vi "List Permanent Variables.vi"(8 "error in (no error)":errorcluster, 11 "CSM-Static-Variable-Manager in":refnum<class "CSM-Static-Variable-Manager.lvclass">) -> (0 "error out":errorcluster, 1 "Permanent Variables":string[](array[string]), 3 "CSM-Static-Variable-Manager out":refnum<class "CSM-Static-Variable-Manager.lvclass">)   [LabVIEW 2017, in "INI-Static-Variable-Support.lvlib" / "CSM-Static-Variable-Manager.lvclass"]
uses:
  CSM-Static-Variable-Manager.lvclass
  CSM-Static-Variable-Manager.lvclass/CSM-Static-Variable-Manager.ctl
  LabVIEW-Config/LabVIEW-Config.lvclass
  <userlib>/_NEVSTOP/Communicable State Machine(CSM)/addons/API-String-Arugments-Support/API String Arguments Support.lvlib
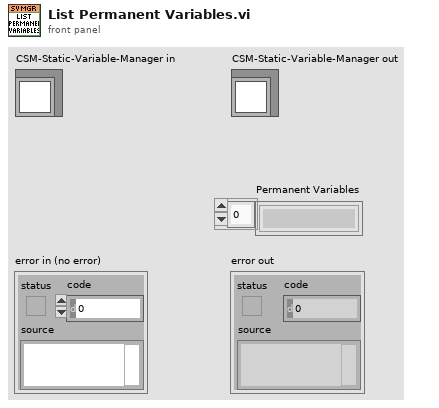
[diagram p1: front panel]
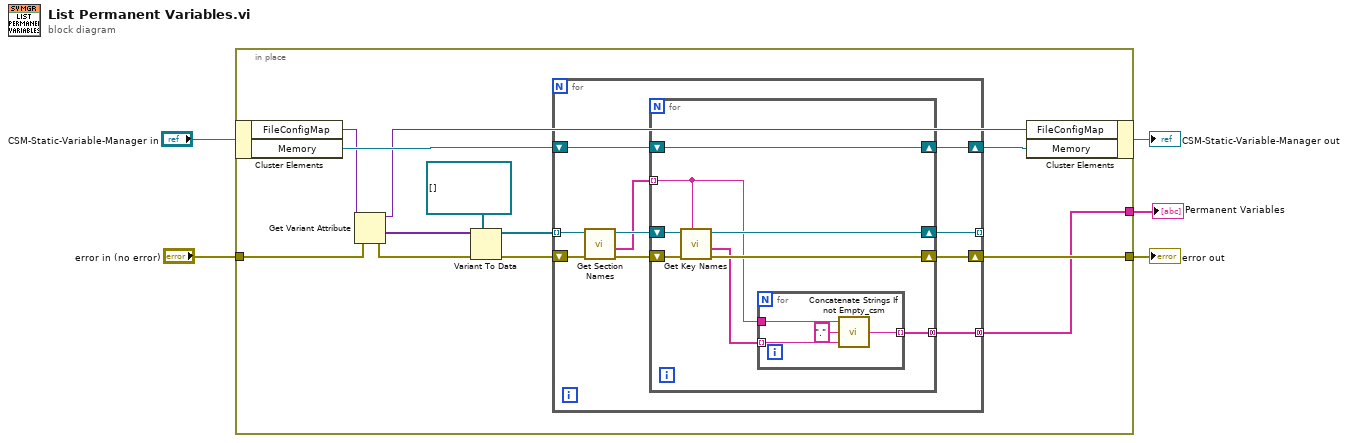
[diagram p0: block diagram]
diagram:
  n1 = in-place {
    in-place-border: "error in (no error)" -> [w12]
    in-place-border: [w8] -> w2
    in-place-border: [w6] -> w1
    n2 = in-place-cluster #1("CSM-Static-Variable-Manager in") -> ("FileConfigMap"=w15:variant, "Memory"=w17:refnum<class "LabVIEW-Config.lvclass">)
    n3 = Get Variant Attribute(Variant=w15, error in=w12) -> (duplicate Variant=w7:variant, values=w14:variant[], error out=w13:errorcluster)  [unwired: 2 in, 1 out]
    n4 = Variant To Data(error in=w13, type=refnum<class "LabVIEW-Config.lvclass">[] [], Variant=w14) -> (data=w9:refnum<class "LabVIEW-Config.lvclass">[], error out=w11:errorcluster)
    n5 = for {
      shift-right: [w25] -> w16
      shift-left: w17 -> [w26]
      shift-right: [w19] -> w8
      shift-left: w11 -> [w23]
      tunnel: w9 -> [w27] mode=indexing
      tunnel: [w20] -> _ mode=indexing
      tunnel: [w18] -> w6 mode=concatenating
      n6 = call "Get Section Names.vi"("error in (no error)"=w23, "Config in"=w27) -> ("error out"=w22:errorcluster, "Section Names"=w21:string[], "Config out"=w24:refnum<class "LabVIEW-Config.lvclass">)  [unwired: 7 in]
      n7 = for {
        shift-right: [w33] -> w25
        shift-left: w26 -> [w33]
        shift-right: [w34] -> w19
        shift-left: w22 -> [w31]
        tunnel: w21 -> [w30] mode=indexing
        shift-right: [w35] -> w20
        shift-left: w24 -> [w32]
        tunnel: [w28] -> w18 mode=concatenating
        n8 = call "Get Key Names.vi"("Section Name"=w30, "error in (no error)"=w31, "Config in"=w32) -> ("error out"=w34:errorcluster, "Key Names"=w29:string[], "Config out"=w35:refnum<class "LabVIEW-Config.lvclass">)  [unwired: 5 in, 1 out]
        n9 = for {
          tunnel: [w39] -> w28 mode=indexing
          tunnel: w29 -> [w38] mode=indexing
          tunnel: w30 -> [w37]
          n10 = call <userlib>:"Concatenate Strings If not Empty_csm.vi"("String"=w38, "seperator(:)"=".", "prefix"=w37) -> ("result"=w39:string)  [unwired: 2 in]
        }
      }
    }
    n11 = in-place-cluster #1("FileConfigMap"=w7, "Memory"=w16) -> (→"CSM-Static-Variable-Manager out":refnum<class "CSM-Static-Variable-Manager.lvclass">)
  }
  "error out" <- w2
  "Permanent Variables" <- w1
